vi "Read Data.vi"(8 "error in":errorcluster, 11 "file path":path) -> (0 "error out":errorcluster, 3 "Data":dbl[][](array[numeric]))   [LabVIEW 2009]
doc: "Reads GPR data from an ASCII file and inverts it."
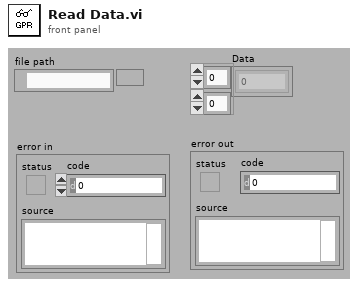
[diagram p1: front panel]
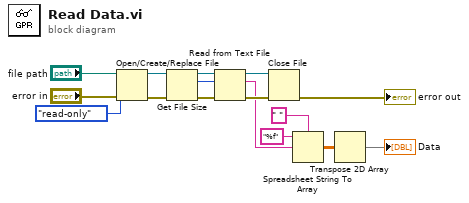
[diagram p0: block diagram]
diagram:
  n1 = Open/Create/Replace File(file path (use dialog)="file path", error in="error in", access (0:read/write)=enum16{"read/write", "read-only", "write-only"}."read-only") -> (refnum out=w4:refnum<file>, error out=w5:errorcluster)  [unwired: 3 in, 1 out]
  n2 = Get File Size(file=w4, error in=w5) -> (refnum out=w7:refnum<file>, size (in bytes)=w6:i64, 0:w8:errorcluster)
  n3 = Read from Text File(file (use dialog)=w7, count=w6, error in=w8) -> (refnum out=w12:refnum<file>, text=w9:string, error out=w11:errorcluster)  [unwired: 1 in, 1 out]
  n4 = Close File(refnum=w12, error in=w11) -> (error out=→"error out":errorcluster)  [unwired: 1 out]
  n5 = Spreadsheet String To Array(delimiter (Tab)=" ", format string="%f", spreadsheet string=w9) -> (array=w14:dbl[][])  [unwired: 1 in]
  n6 = Transpose 2D Array(2D array=w14) -> (transposed array=→"Data":dbl[][])
